vi "meTEC_Set_ID 2000_Input Selection.vi"(6 "Instance (1)":u8=1, 8 "error in (no error)":errorcluster, 9 "TEC Configuration_IN":T1={"VISA resource name"="", "Device Address"=2}, 10 "Sequence No.":u16=5552, 11 "Input Selection (ID 2000)":i32=2 min=0 max=2 step=1) -> (0 "error out":errorcluster, 1 "TEC Configuration_OUT":T1={"VISA resource name"="", "Device Address"=2}, 3 "Serial Message_Read":string)   [LabVIEW 2023]
uses:
  TypeDefs/meTEC_Configuration.ctl
panel:
  # "--- Inputs ---"
  # "--- Outputs ---"
  # "0: Static Current/Voltage (Uses ID 2020...)\n1: Live Current/Voltage (Uses ID 50001...)\n2: Temperature Controller"
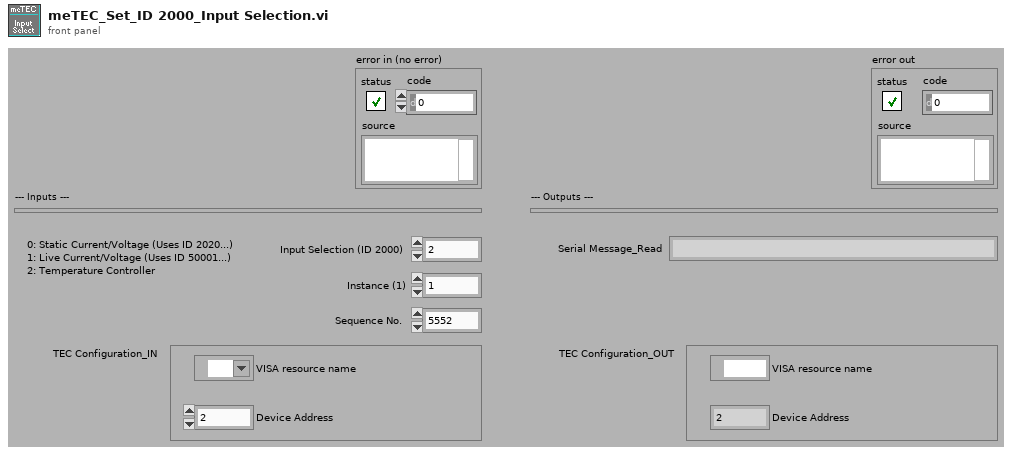
[diagram p1: front panel]
types:
  T1 = typedef "meTEC_Configuration.ctl" = cluster{"VISA resource name":refnum<visa-resource-name>, "Device Address":u16}
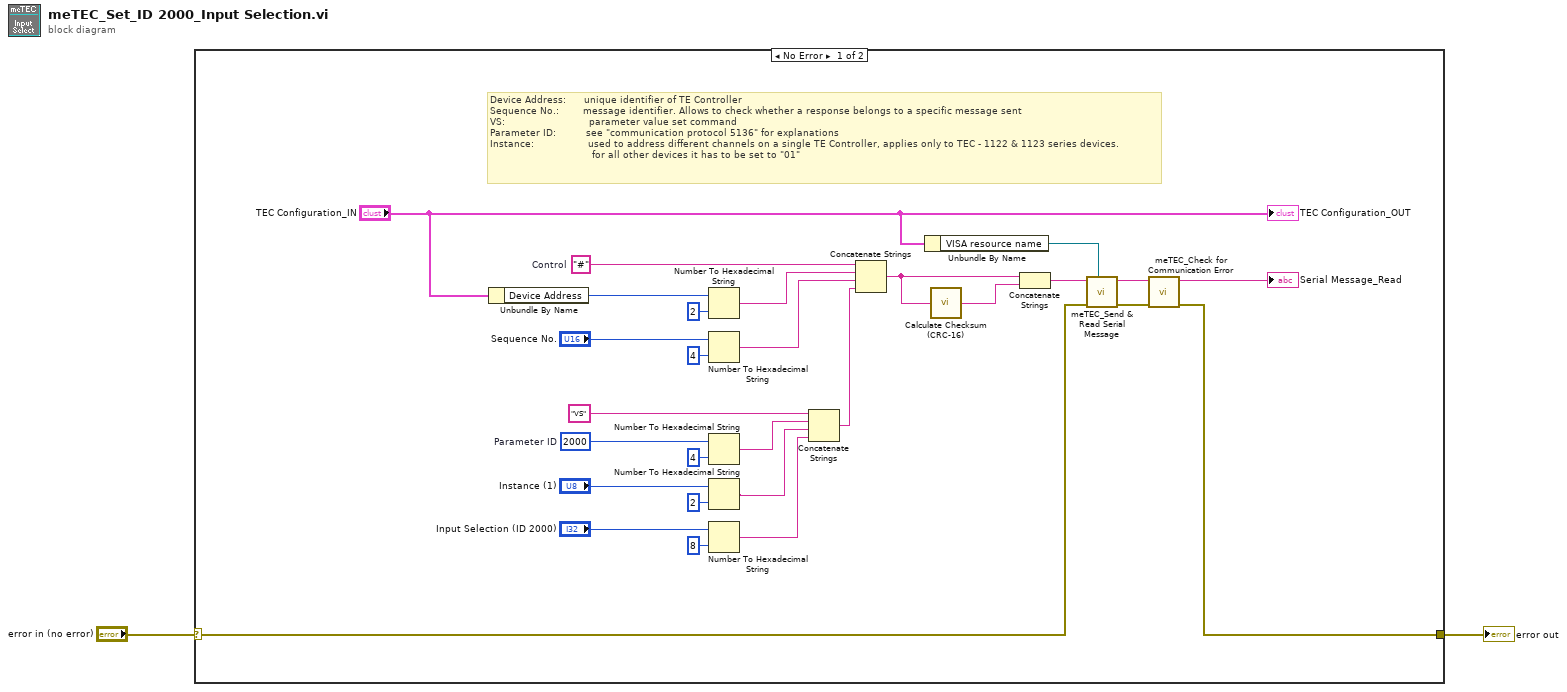
[diagram p0: block diagram]
diagram:
  n1 = case shown="No Error" "error in (no error)" {
    selector: "error in (no error)" -> [w16 w31]
    tunnel: [w5 w31] -> w2
    frame No Error {
      w24 = "#"  # Control
      w29 = 2000  # Parameter ID
      # "Device Address:      unique identifier of TE Controller\nSequence No.:        message identifier. Allows to check whether a response belongs to a specific message sent \nVS:                            parameter value set command\nParameter ID:          see \"communication protocol 5136\" for explanations\nInstance:                  used to address different channels on a single TE Controller, applies only to TEC - 1122 & 1123 series devices.\n                                  for all other devices it has to be set to \"01\""
      n2 = Unbundle By Name("TEC Configuration_IN") -> ("Device Address"=w11:u16)
      n3 = Number To Hexadecimal String(1:i16 2 ("width (-)"), 2:w11) -> (0:w19:string)
      n4 = Number To Hexadecimal String(1:i16 4 ("width (-)"), 2:"Sequence No.") -> (0:w23:string)
      n5 = Number To Hexadecimal String(1:i16 4 ("width (-)"), 2:w29) -> (0:w27:string)
      n6 = Number To Hexadecimal String(1:i16 2 ("width (-)"), 2:"Instance (1)") -> (0:w12:string)
      n7 = Number To Hexadecimal String(1:i16 8 ("width (-)"), 2:"Input Selection (ID 2000)") -> (0:w8:string)
      n8 = Concatenate Strings("VS", w27, w12, w8) -> (w18:string)
      n9 = Concatenate Strings(w24, w19, w23, w18) -> (w22:string)
      n10 = Unbundle By Name("TEC Configuration_IN") -> ("VISA resource name"=w14:refnum<visa-resource-name>)
      n11 = call "Calculate Checksum (CRC-16).vi"("Message"=w22) -> ("CRC [String]"=w21:string)  [unwired: 1 in]
      n12 = Concatenate Strings(w22, w21) -> (w17:string)
      n13 = call "meTEC_Send & Read Serial Message.vi"("VISA resource name"=w14, "error in (no error)"=w16, "Serial Message"=w17) -> ("error out"=w15:errorcluster, "Serial Message_Read"=w4:string)  [unwired: 7 in]
      n14 = call "meTEC_Check for Communication Error.vi"("error in (no error)"=w15, "Serial Message_IN"=w4) -> ("error out"=w5:errorcluster, "Serial Message_OUT"=→"Serial Message_Read":string)  [unwired: 8 in]
      "TEC Configuration_OUT" <- "TEC Configuration_IN"
    }
    frame Error {
    }
  }
  "error out" <- w2
